vi "Is Pin Array Valid.vi"(11 "pin or relay names":string[](array[string])) -> (3 "valid":bool)   [LabVIEW 2020, in "Plug-In SDK Measurement.lvlib" / "Measure Call Context.lvclass"]
uses:
  Measure Call Context.lvclass
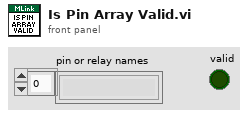
[diagram p1: front panel]
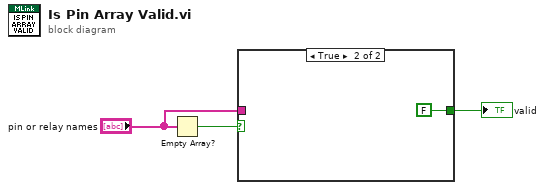
[diagram p0: block diagram]
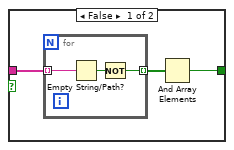
[diagram p2: hidden frame]
diagram:
  n1 = Empty Array?(array="pin or relay names") -> (empty?=w3:bool)
  n2 = case shown="True" w3 {
    tunnel: [w4 FALSE] -> w2
    tunnel: "pin or relay names" -> [w6 _]
    frame False {
      n3 = for {
        tunnel: w6 -> [w9] mode=indexing
        tunnel: [w7] -> w5 mode=indexing
        n4 = Empty String/Path?(string/path=w9) -> (empty?=w8:bool)
        n5 = Not(x=w8) -> (.not. x?=w7:bool)
      }
      n6 = And Array Elements(Boolean array=w5) -> (logical AND=w4:bool)
    }
    frame True {
    }
  }
  "valid" <- w2
